vi "32xx_Write_String_COM.vi"(7 "Chaîne à écrire":string="0 VOLT MES\r" caption="String to Write", 8 "entrée d'erreur":errorcluster caption="entrée d'erreur (pas d'erreur)", 11 "Port d'entrée":refnum<visa-resource-name>="COM1") -> (0 "sortie d'erreur":errorcluster, 3 "Port de sortie":refnum<visa-resource-name>="COM1")   [LabVIEW 2020]
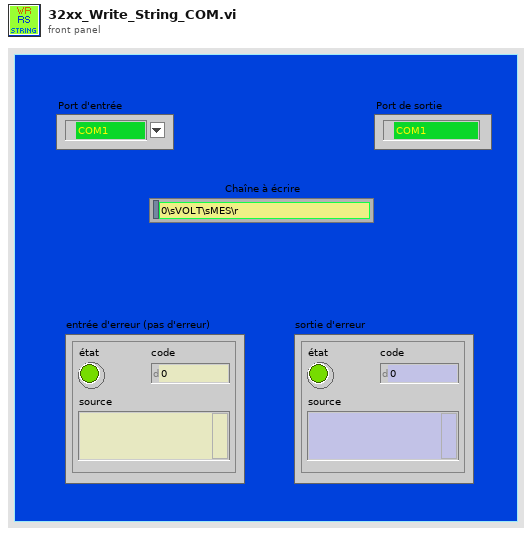
[diagram p1: front panel]
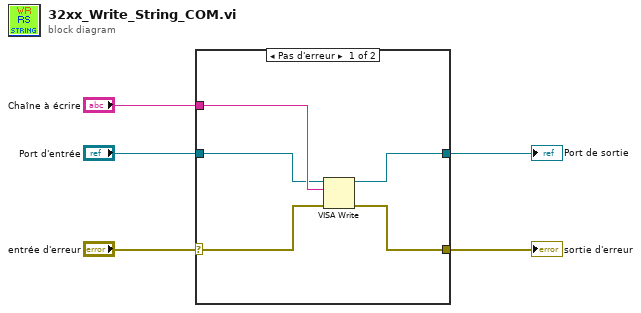
[diagram p0: block diagram]
diagram:
  n1 = case shown="Pas d'erreur" "entrée d'erreur" {
    selector: "entrée d'erreur" -> [w6 w11]
    tunnel: "Chaîne à écrire" -> [w10 _]
    tunnel: "Port d'entrée" -> [w9 w12]
    tunnel: [w8 w11] -> w3
    tunnel: [w7 w12] -> w2
    frame No Error {
      n2 = VISA Write(VISA resource name=w9, write buffer=w10, error in (no error)=w6) -> (VISA resource name out=w7:refnum<visa-resource-name>, error out=w8:errorcluster)  [unwired: 1 out]
    }
    frame Error {
    }
  }
  "Port de sortie" <- w2
  "sortie d'erreur" <- w3
